vi "FT_Get_Number_of_Devices2011.vi"() -> (0 "Number of Devices":u16, 1 "FT_Status":u32(ring) items=["FT_OK", "FT_INVALID_HANDLE", "FT_DEVICE_NOT_FOUND", "FT_DEVICE_NOT_OPENED", "FT_IO_ERROR", "FT_INSUFFICIENT_RESOURCES", "FT_INVALID_PARAMETER", "FT_INVALID_BAUD_RATE", "FT_DEVICE_NOT_OPENED_FOR_ERASE", "FT_DEVICE_NOT_OPENED_FOR_WRITE", "FT_FAILED_TO_WRITE_DEVICE", "FT_EEPROM_READ_FAILED", "FT_EEPROM_WRITE_FAILED", "FT_EEPROM_ERASE_FAILED", "FT_EEPROM_NOT_PRESENT", "FT_EEPROM_NOT_PROGRAMMED", "FT_INVALID_ARGS", "FT_NOT_SUPPORTED", "FT_OTHER_ERROR"])   [LabVIEW 2017]
uses:
  FTD2XX.dll
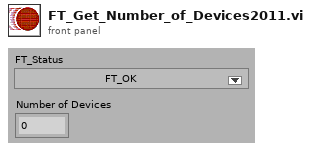
[diagram p1: front panel]
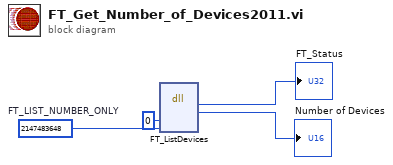
[diagram p0: block diagram]
diagram:
  w2 = u32 2147483648  # FT_LIST_NUMBER_ONLY
  n1 = dll-call lib="FTD2XX.dll" fn="FT_ListDevices" label="FT_List_Devices"(u32 0 ("input param"), "Flags"=w2) -> ("FT_Status"=→"FT_Status":u32, →"Number of Devices":u32)  [unwired: 6 in, 2 out]
